vi "Get Exclusive Subsystems.vi"(8 "error in (no error)":errorcluster, 10 "Subsystem Array B":T1[](array[typedef]), 11 "Subsystem Array A":T1[](array[typedef])) -> (0 "error out":errorcluster, 2 "Exist?":bool, 3 "Exclusive Subsystems":T1[](array[typedef]))   [LabVIEW 2024]
doc: "Returns subsystems that exist in the array B but not in the array A."
uses:
  Controls/Server/Subsystem Configuration.ctl
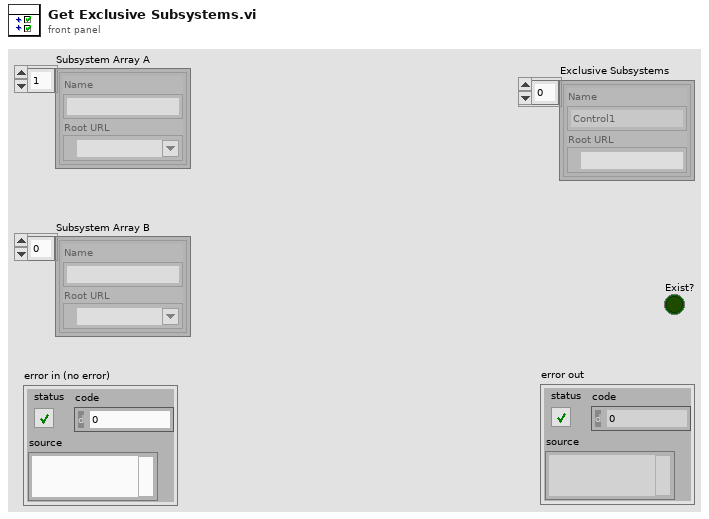
[diagram p1: front panel]
types:
  T1 = typedef "Subsystem Configuration.ctl" = cluster{"Name":string, "Root URL":refnum<k21>}
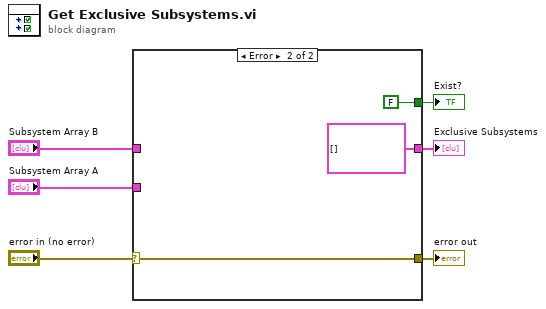
[diagram p0: block diagram]
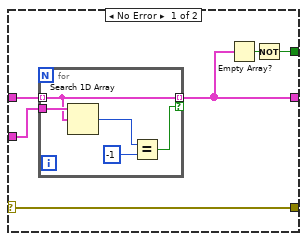
[diagram p2: hidden frame]
diagram:
  n1 = case shown="Error" "error in (no error)" {
    selector: "error in (no error)" -> [w12 w20]
    tunnel: [w12 w20] -> w5
    tunnel: [w7 FALSE] -> w4
    tunnel: [w9 T1[] []] -> w3
    tunnel: "Subsystem Array B" -> [w11 _]
    tunnel: "Subsystem Array A" -> [w10 _]
    frame No Error {
      n2 = for {
        tunnel: w10 -> [w17]
        tunnel: w11 -> [w16] mode=indexing
        tunnel: [w16] -> w9 mode=indexing if=w15
        n3 = Search 1D Array(1D array=w17, element=w16) -> (index of element=w14:i32)  [unwired: 1 in]
        n4 = Equal?(x=w14, y=-1 ("x")) -> (x = y?=w15:bool)
      }
      n5 = Empty Array?(array=w9) -> (empty?=w8:bool)
      n6 = Not(x=w8) -> (.not. x?=w7:bool)
    }
    frame Error {
    }
  }
  "error out" <- w5
  "Exist?" <- w4
  "Exclusive Subsystems" <- w3
